vi "Read head.vi"(8 "error in (no error)":errorcluster, 11 "DoublyLinkedList in":refnum<class "DoublyLinkedList.lvclass">) -> (0 "error out":errorcluster, 2 "DoublyNodeRef.lvclass":refnum<class "Iterator.lvclass">, 3 "DoublyLinkedList out":refnum<class "DoublyLinkedList.lvclass">)   [LabVIEW 2021, in "DoublyLinkedList.lvclass"]
uses:
  DoublyLinkedList.lvclass
  Iterator/Iterator.lvclass
  DoublyLinkedList.lvclass/DoublyLinkedList.ctl
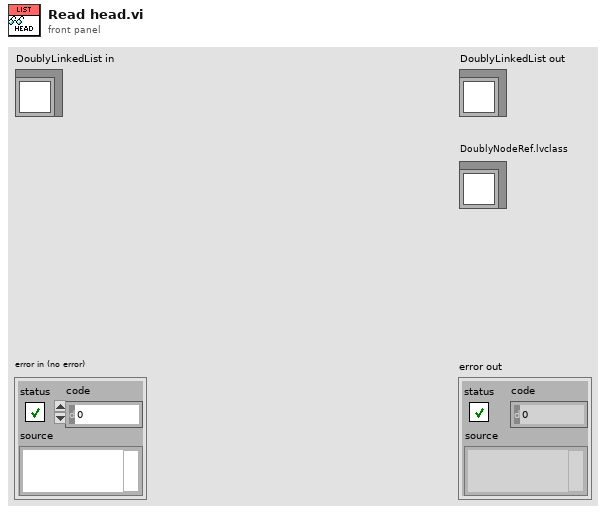
[diagram p1: front panel]
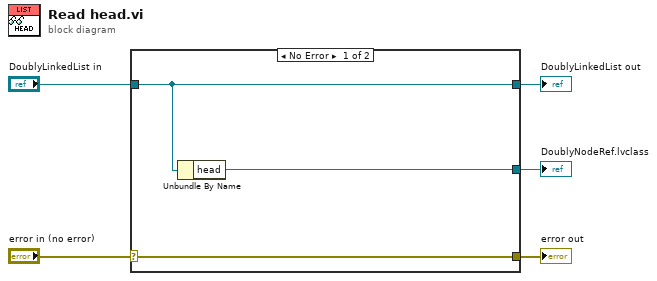
[diagram p0: block diagram]
diagram:
  n1 = case shown="No Error" "error in (no error)" {
    selector: "error in (no error)" -> [w8 w9]
    tunnel: [w8 w9] -> w4
    tunnel: [w7 w10] -> w2
    tunnel: "DoublyLinkedList in" -> [w7 w10]
    tunnel: [w6 _] -> w1
    frame No Error {
      n2 = Unbundle By Name(w7) -> ("head"=w6:refnum<class "Iterator.lvclass">)
    }
    frame Error {
    }
  }
  "error out" <- w4
  "DoublyLinkedList out" <- w2
  "DoublyNodeRef.lvclass" <- w1
